vi "soap_labview.vi"() -> ()   [LabVIEW 2021]
uses:
  <vilib>/numeric/Random Number (Range) U64.vi
  <vilib>/numeric/sub_Random U32.vi
panel:
  out "DATA PANEL":T1
  out "DISPATCH 3":bool
  out "DISPATCH 2":bool
  out "DISPATCH":bool
  out "Coconut Oil/metreic Ton":string
  out "Olive oil/metric Ton":string
  out "STATION 3":u8(slide) scale=0.0..2.0
  out "STATION 2":u8(slide) scale=0.0..2.0
  out "STATION 1":u8(slide) scale=0.0..2.0
  out "PACKAGING":bool
  out "STAMPING":bool
  out "CUTTING":bool
  out "REST TIME":dbl(knob) scale=0.0..12.0
  out "Maintianed temperature":dbl(slide) scale=70.0..110.0
  out "STRAWBERRY":bool
  out "LAVENDER":bool
  out "ROSE":bool
  out "CSTR":bool
  out "MIXING TIME":dbl(knob) scale=0.0..4.0
  out "Maintained temperature":dbl(slide) scale=0.0..130.0
  out "Water":bool
  out "SEA SALT":bool
  out "SODIUM HYDROXIDE(NaOH)":bool
  out "SOFT OIL":bool
  out "HARD FATS":bool
  out "LAURIC OILS":bool
  out "TEMPS":dbl
  out "TEMPL":dbl
  out "TEMPR":dbl
  out "number":u64
  out "index of element":i32
  out "STRAWBERRYN":dbl
  out "LAVENDARN":dbl
  in  "Variable":dbl
  out "ROSEN":dbl
  out "TOTAL NUMBER OF EVENTS":i32
  out "OIL PROCESS":string
  out "PROCESS":string
  # "SOAP MANUFACTURING PROCESS"
  # "CONTINUOUS STIRRED TANK REACTOR"
  # "COOLING PROCESS"
  # "STATION"
  # "RAW MATERIAL PROCESS"
  # "OIL"
  # "CUTTING"
  # "LYE"
  # "STAMPING"
  # "BRINE"
  # "WATER"
  # "USD"
  # "USD"
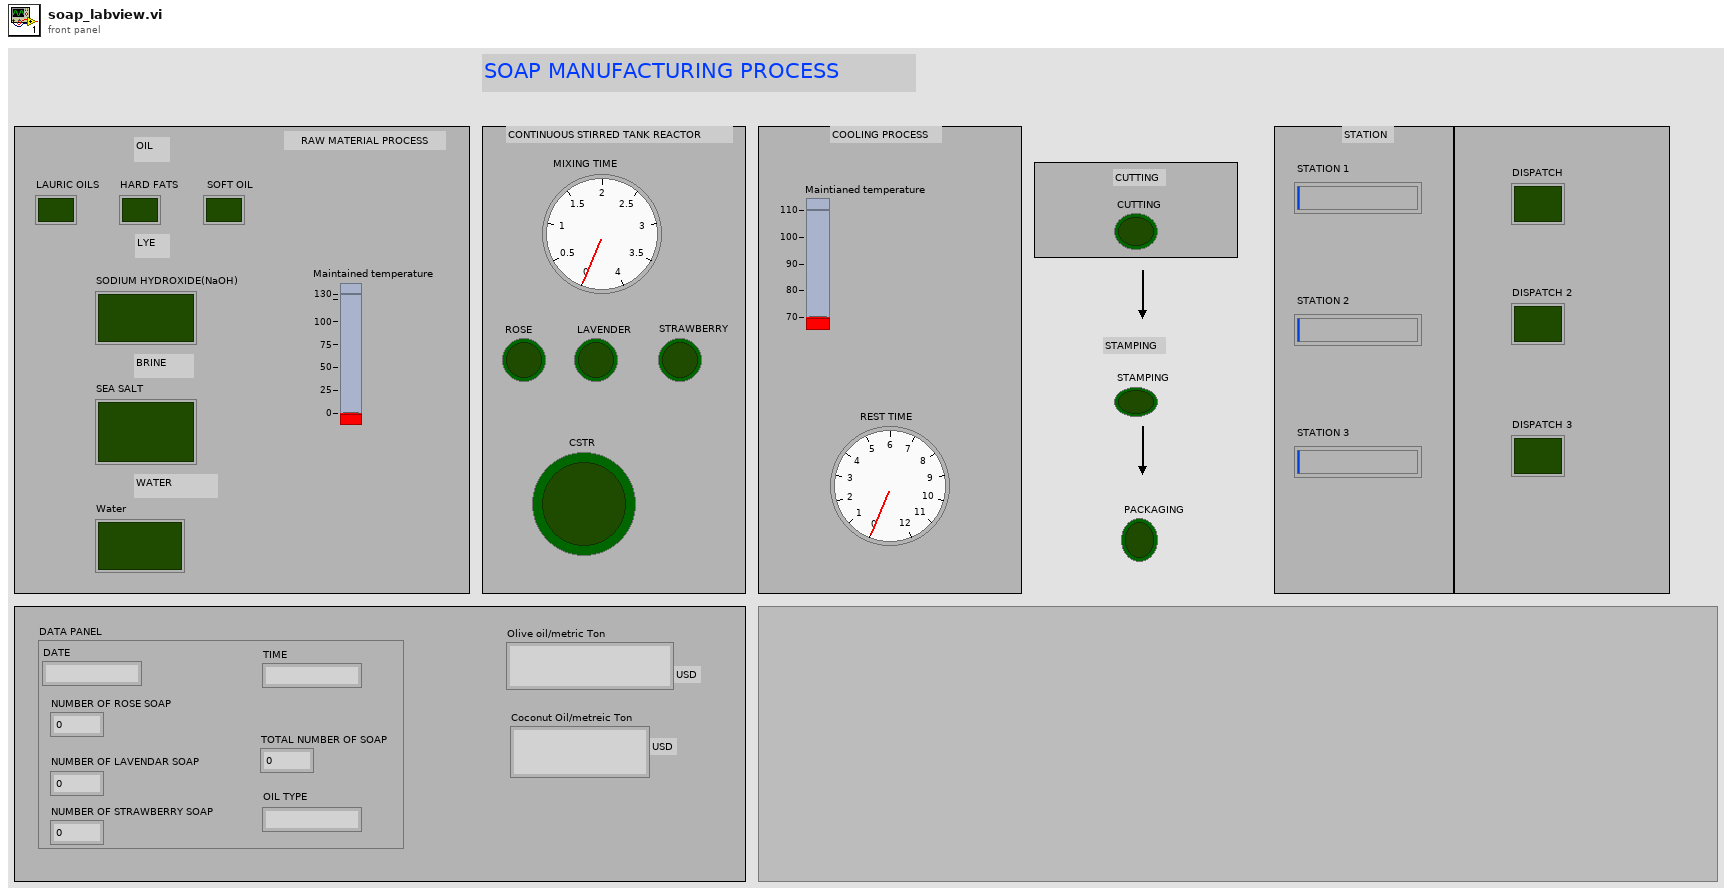
[diagram p1: front panel]
types:
  T1 = cluster{"DATE":string, "TIME":string, "NUMBER OF ROSE SOAP":dbl, "NUMBER OF LAVENDAR SOAP":dbl, "NUMBER OF STRAWBERRY SOAP":dbl, "TOTAL NUMBER OF SOAP":dbl, "OIL TYPE":string}
  T2 = cluster{"date string":string, "time string":string, "ROSEN":dbl, "LAVENDARN":dbl, "STRAWBERRYN":dbl, "TOTAL NUMBER OF EVENTS":i32, "OIL PROCESS":string}
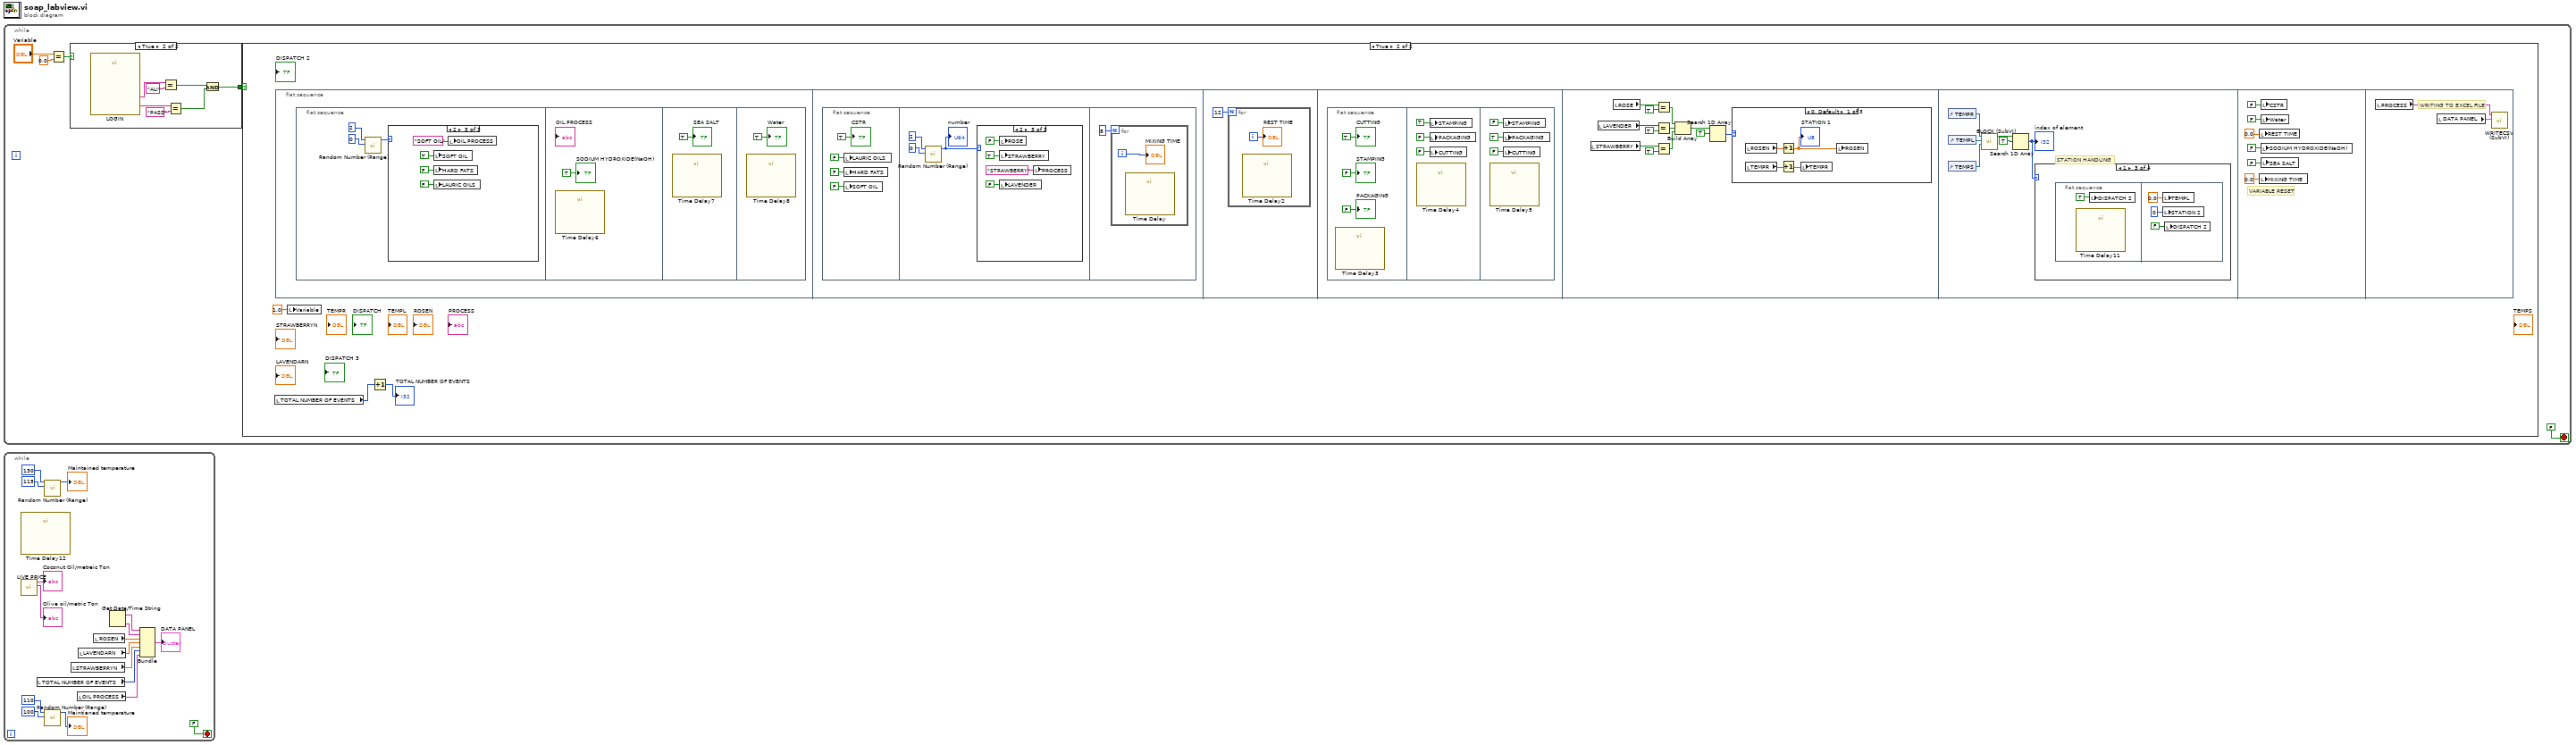
[diagram p0: block diagram]
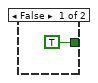
[diagram p2: hidden frame]
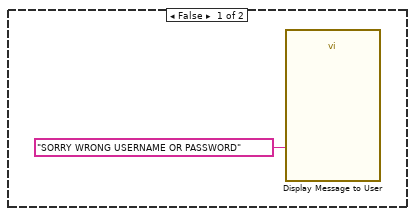
[diagram p3: hidden frame]
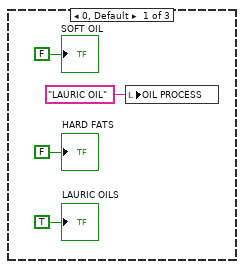
[diagram p4: hidden frame]
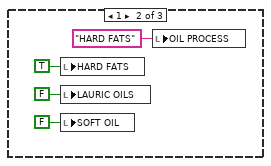
[diagram p5: hidden frame]
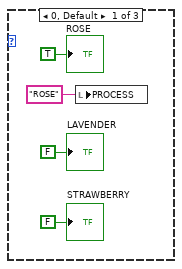
[diagram p6: hidden frame]
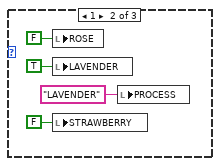
[diagram p7: hidden frame]
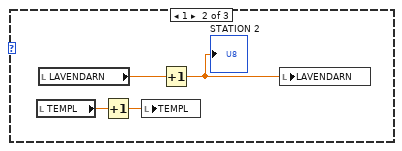
[diagram p8: hidden frame]
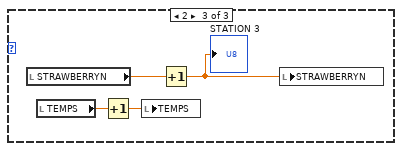
[diagram p9: hidden frame]
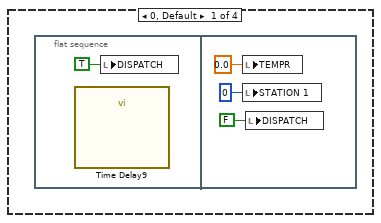
[diagram p10: hidden frame]
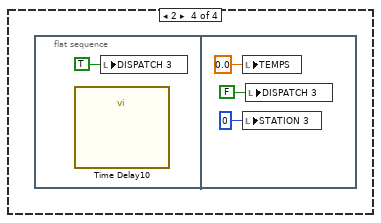
[diagram p12: hidden frame]
diagram:
  n1 = while {
    stop <- FALSE stop-if-true
    n2 = Equal?(x="Variable", y=0.0) -> (x = y?=w1:bool)
    n3 = case shown="True" w1 {
      tunnel: [TRUE w7] -> w4
      frame False {
      }
      frame True {
        n4 = call "LOGIN"() -> ("PASSWORD"=w11:string, "NAME"=w10:string)  [unwired: 16 in, 2 out]
        n5 = Equal?(x=w10, y="ALI") -> (x = y?=w13:bool)
        n6 = Equal?(x=w11, y="PASS") -> (x = y?=w12:bool)
        n7 = And(x=w13, y=w12) -> (x .and. y?=w7:bool)
      }
    }
    n8 = case shown="True" w4 {
      frame False {
        n9 = call "Display Message to User"("Message"="SORRY WRONG USERNAME OR PASSWORD") -> ()  [unwired: 9 in, 2 out]
      }
      frame True {
        n10 = local read "TOTAL NUMBER OF EVENTS"() -> (w15:i32)
        n11 = flat-sequence {
          frame #0 {
            n12 = flat-sequence {
              frame #0 {
                n13 = call-poly <vilib>:"Random Number (Range).vi"("lower bound (0)"=u64 0, "upper bound (100)"=u64 2) -> ("number"=w18:u64)  [unwired: 9 in]
                n14 = case shown="2" w18 {
                  frame 0, Default {
                    n15 = local write "OIL PROCESS"("LAURIC OIL" ("OIL PROCESS")) -> ()
                    "LAURIC OILS" <- TRUE ("LAURIC OILS")
                    "HARD FATS" <- FALSE ("HARD FATS")
                    "SOFT OIL" <- FALSE ("SOFT OIL")
                  }
                  frame 1 {
                    n16 = local write "HARD FATS"(TRUE ("HARD FATS")) -> ()
                    n17 = local write "LAURIC OILS"(FALSE ("LAURIC OILS")) -> ()
                    n18 = local write "SOFT OIL"(FALSE ("SOFT OIL")) -> ()
                    n19 = local write "OIL PROCESS"("HARD FATS" ("OIL PROCESS")) -> ()
                  }
                  frame 2 {
                    n20 = local write "SOFT OIL"(TRUE ("SOFT OIL")) -> ()
                    n21 = local write "HARD FATS"(FALSE ("HARD FATS")) -> ()
                    n22 = local write "LAURIC OILS"(FALSE ("LAURIC OILS")) -> ()
                    n23 = local write "OIL PROCESS"("SOFT OIL" ("OIL PROCESS")) -> ()
                  }
                }
              }
              frame #1 {
                n24 = call "Time Delay6"() -> ()  [unwired: 11 in, 1 out]
                "SODIUM HYDROXIDE(NaOH)" <- TRUE ("SODIUM HYDROXIDE(NaOH)")
              }
              frame #2 {
                n25 = call "Time Delay7"() -> ()  [unwired: 11 in, 1 out]
                "SEA SALT" <- TRUE ("SEA SALT")
              }
              frame #3 {
                n26 = call "Time Delay8"() -> ()  [unwired: 11 in, 1 out]
                "Water" <- TRUE ("Water")
              }
            }
          }
          frame #1 {
            n27 = flat-sequence {
              frame #0 {
                n28 = local write "LAURIC OILS"(FALSE ("LAURIC OILS")) -> ()
                n29 = local write "HARD FATS"(FALSE ("HARD FATS")) -> ()
                n30 = local write "SOFT OIL"(FALSE ("SOFT OIL")) -> ()
                "CSTR" <- TRUE ("CSTR")
              }
              frame #1 {
                n31 = call-poly <vilib>:"Random Number (Range).vi"("lower bound (0)"=u64 0, "upper bound (100)"=u64 2) -> ("number"=w40:u64)  [unwired: 9 in]
                "number" <- w40
                n32 = case shown="2" w40 {
                  frame 0, Default {
                    n33 = local write "PROCESS"("ROSE" ("PROCESS")) -> ()
                    "ROSE" <- TRUE ("ROSE")
                    "LAVENDER" <- FALSE ("LAVENDER")
                    "STRAWBERRY" <- FALSE ("STRAWBERRY")
                  }
                  frame 1 {
                    n34 = local write "ROSE"(FALSE ("SOFT OIL")) -> ()
                    n35 = local write "LAVENDER"(TRUE ("LAVENDER")) -> ()
                    n36 = local write "STRAWBERRY"(FALSE ("STRAWBERRY")) -> ()
                    n37 = local write "PROCESS"("LAVENDER" ("PROCESS")) -> ()
                  }
                  frame 2 {
                    n38 = local write "ROSE"(FALSE ("ROSE")) -> ()
                    n39 = local write "STRAWBERRY"(TRUE ("STRAWBERRY")) -> ()
                    n40 = local write "LAVENDER"(FALSE ("LAVENDER")) -> ()
                    n41 = local write "PROCESS"("STRAWBERRY" ("PROCESS")) -> ()
                  }
                }
              }
              frame #2 {
                n42 = for {
                  N: 8 -> [_]
                  i -> [w56]
                  n43 = call "Time Delay"() -> ()  [unwired: 11 in, 1 out]
                  "MIXING TIME" <- w56
                }
              }
            }
          }
          frame #2 {
            n44 = for {
              N: 12 -> [_]
              i -> [w58]
              n45 = call "Time Delay2"() -> ()  [unwired: 11 in, 1 out]
              "REST TIME" <- w58
            }
          }
          frame #3 {
            n46 = flat-sequence {
              frame #0 {
                n47 = call "Time Delay3"() -> ()  [unwired: 11 in, 1 out]
                "CUTTING" <- TRUE ("CUTTING")
                "STAMPING" <- FALSE ("STAMPING")
                "PACKAGING" <- FALSE ("PACKAGING")
              }
              frame #1 {
                n48 = call "Time Delay4"() -> ()  [unwired: 11 in, 1 out]
                n49 = local write "STAMPING"(TRUE ("STAMPING")) -> ()
                n50 = local write "PACKAGING"(FALSE ("PACKAGING")) -> ()
                n51 = local write "CUTTING"(FALSE ("CUTTING")) -> ()
              }
              frame #2 {
                n52 = call "Time Delay5"() -> ()  [unwired: 11 in, 1 out]
                n53 = local write "STAMPING"(FALSE ("STAMPING")) -> ()
                n54 = local write "PACKAGING"(TRUE ("PACKAGING")) -> ()
                n55 = local write "CUTTING"(FALSE ("CUTTING")) -> ()
              }
            }
          }
          frame #4 {
            n56 = local read "STRAWBERRY"() -> (w74:bool)
            n57 = local read "LAVENDER"() -> (w76:bool)
            n58 = local read "ROSE"() -> (w79:bool)
            n59 = Equal?(x=w79, y=TRUE) -> (x = y?=w77:bool)
            n60 = Equal?(x=w76, y=TRUE) -> (x = y?=w72:bool)
            n61 = Equal?(x=w74, y=TRUE) -> (x = y?=w71:bool)
            n62 = Build Array(w77, w72, w71) -> (w70:bool[])
            n63 = Search 1D Array(1D array=w70, element=TRUE) -> (index of element=w68:i32)  [unwired: 1 in]
            n64 = case shown="0, Default" w68 {
              frame 0, Default {
                n65 = local read "ROSEN"() -> (w83:dbl)
                n66 = local read "TEMPR"() -> (w81:dbl)
                n67 = Increment(x=w83) -> (x+1=w82:dbl)
                "STATION 1" <- w82
                n68 = Increment(x=w81) -> (x+1=w80:dbl)
                n69 = local write "TEMPR"(w80) -> ()
                n70 = local write "ROSEN"(w82) -> ()
              }
              frame 1 {
                n71 = local read "TEMPL"() -> (w85:dbl)
                n72 = local read "LAVENDARN"() -> (w87:dbl)
                n73 = Increment(x=w85) -> (x+1=w84:dbl)
                n74 = local write "TEMPL"(w84) -> ()
                n75 = Increment(x=w87) -> (x+1=w86:dbl)
                "STATION 2" <- w86
                n76 = local write "LAVENDARN"(w86) -> ()
              }
              frame 2 {
                n77 = local read "STRAWBERRYN"() -> (w91:dbl)
                n78 = local read "TEMPS"() -> (w89:dbl)
                n79 = Increment(x=w89) -> (x+1=w88:dbl)
                n80 = local write "TEMPS"(w88) -> ()
                n81 = Increment(x=w91) -> (x+1=w90:dbl)
                "STATION 3" <- w90
                n82 = local write "STRAWBERRYN"(w90) -> ()
              }
            }
          }
          frame #5 {
            # "STATION HANDLING"
            n83 = control-ref of="TEMPR"() -> (w94:refnum<vi>)
            n84 = control-ref of="TEMPL"() -> (w93:refnum<vi>)
            n85 = control-ref of="TEMPS"() -> (w92:refnum<vi>)
            n86 = call "BLOCK (SubVI).vi"("reference 3"=w92, "reference in"=w93, "Digital in"=w94) -> ("Array"=w97:bool[])  [unwired: 8 in]
            n87 = Search 1D Array(1D array=w97, element=TRUE) -> (index of element=w95:i32)  [unwired: 1 in]
            "index of element" <- w95
            n88 = case shown="1" w95 {
              frame 0, Default {
                n89 = flat-sequence {
                  frame #0 {
                    n90 = call "Time Delay9"() -> ()  [unwired: 11 in, 1 out]
                    n91 = local write "DISPATCH"(TRUE ("DISPATCH")) -> ()
                  }
                  frame #1 {
                    n92 = local write "TEMPR"(0.0 ("TEMPR")) -> ()
                    n93 = local write "STATION 1"(u8 0 ("STATION 1")) -> ()
                    n94 = local write "DISPATCH"(FALSE ("DISPATCH")) -> ()
                  }
                }
              }
              frame -1 {
              }
              frame 1 {
                n95 = flat-sequence {
                  frame #0 {
                    n96 = call "Time Delay11"() -> ()  [unwired: 11 in, 1 out]
                    n97 = local write "DISPATCH 2"(TRUE ("DISPATCH 2")) -> ()
                  }
                  frame #1 {
                    n98 = local write "TEMPL"(0.0 ("TEMPL")) -> ()
                    n99 = local write "STATION 2"(u8 0 ("STATION 2")) -> ()
                    n100 = local write "DISPATCH 2"(FALSE ("DISPATCH 2")) -> ()
                  }
                }
              }
              frame 2 {
                n101 = flat-sequence {
                  frame #0 {
                    n102 = call "Time Delay10"() -> ()  [unwired: 11 in, 1 out]
                    n103 = local write "DISPATCH 3"(TRUE ("DISPATCH 3")) -> ()
                  }
                  frame #1 {
                    n104 = local write "TEMPS"(0.0 ("TEMPS")) -> ()
                    n105 = local write "STATION 3"(u8 0 ("STATION 3")) -> ()
                    n106 = local write "DISPATCH 3"(FALSE ("DISPATCH 3")) -> ()
                  }
                }
              }
            }
          }
          frame #6 {
            # "VARIABLE RESET"
            n107 = local write "REST TIME"(0.0 ("REST TIME")) -> ()
            n108 = local write "MIXING TIME"(0.0 ("MIXING TIME")) -> ()
            n109 = local write "CSTR"(FALSE ("CSTR")) -> ()
            n110 = local write "Water"(FALSE ("Water")) -> ()
            n111 = local write "SODIUM HYDROXIDE(NaOH)"(FALSE ("SODIUM HYDROXIDE(NaOH)")) -> ()
            n112 = local write "SEA SALT"(FALSE ("SEA SALT")) -> ()
          }
          frame #7 {
            # "WRITING TO EXCEL FILE"
            n113 = local read "PROCESS"() -> (w116:string)
            n114 = local read "DATA PANEL"() -> (w117:T1)
            n115 = call "WRITECSV (SubVI).vi"("DATA PANEL"=w117, "PROCESS"=w116) -> ()  [unwired: 10 in]
          }
        }
        n116 = local write "Variable"(1.0 ("Variable")) -> ()
        n117 = Increment(x=w15) -> (x+1=→"TOTAL NUMBER OF EVENTS":i32)
      }
    }
  }
  n118 = while {
    stop <- FALSE stop-if-true
    n119 = call "LIVE PRICE.vi"() -> ("String 2"=→"Olive oil/metric Ton":string, "String"=→"Coconut Oil/metreic Ton":string)  [unwired: 10 in]
    n120 = call "Time Delay12"() -> ()  [unwired: 11 in, 1 out]
    n121 = local read "TOTAL NUMBER OF EVENTS"() -> (w120:i32)
    n122 = call-poly <vilib>:"Random Number (Range).vi"("lower bound (0)"=u64 115, "upper bound (100)"=u64 130) -> ("number"=→"Maintained temperature":u64)  [unwired: 9 in]
    n123 = call-poly <vilib>:"Random Number (Range).vi"("lower bound (0)"=u64 100, "upper bound (100)"=u64 110) -> ("number"=→"Maintianed temperature":u64)  [unwired: 9 in]
    n124 = local read "STRAWBERRYN"() -> (w121:dbl)
    n125 = local read "OIL PROCESS"() -> (w118:string)
    n126 = local read "LAVENDARN"() -> (w122:dbl)
    n127 = local read "ROSEN"() -> (w123:dbl)
    n128 = Get Date/Time String() -> (date string=w125:string, time string=w124:string)  [unwired: 3 in]
    n129 = Bundle("date string"=w125, "time string"=w124, "ROSEN"=w123, "LAVENDARN"=w122, "STRAWBERRYN"=w121, "TOTAL NUMBER OF EVENTS"=w120, "OIL PROCESS"=w118) -> (→"DATA PANEL":T2)  [unwired: 1 in]
  }
